vi "Channel Initialize.vi"(0 "Item Ref in":T2 format="%.0x", 7 "error in (no error)":errorcluster, 8 "Starting Address Ref in":refnum<vi>) -> (14 "Default Value":dbl, 16 "Radix":T1, 17 "Sub-Index (Bool)":u16, 18 "Registers":i32, 19 "input?":bool, 20 "Channel Ref out":T2 format="%.0x", 21 "Name":string, 22 "Description":string, 23 "Starting Address":u16, 24 "DataType":T3, 25 "Valid?":bool, 26 "Status Message":string, 27 "error out":errorcluster)   [LabVIEW 2019, in "Modbus Master System Explorer.lvlib"]
uses:
  Modbus Master System Explorer.lvlib
  Shared/Controls/Data Model/DataType.ctl
  <vilib>/NI VeriStand/Custom Device API/Custom Device Item Ref.ctl
  Radix.ctl
  <vilib>/NI VeriStand/Custom Device API/Custom Device API.lvlib
  Shared/Modbus Master Shared.lvlib
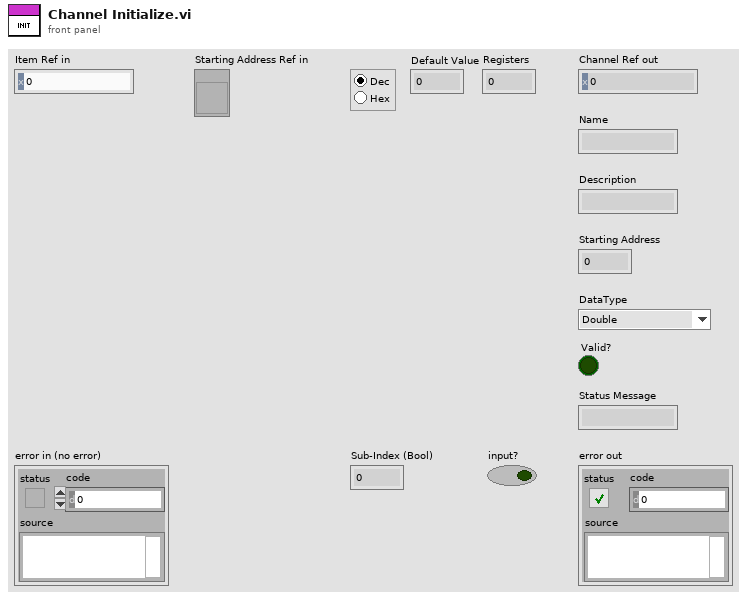
[diagram p1: front panel]
types:
  T1 = typedef "Modbus Master System Explorer.lvlib/Radix.ctl" = enum32{"Decimal", "Hexidecimal"}
  T2 = typedef "Custom Device API.lvlib/Custom Device Item Ref.ctl" = u64
  T3 = typedef "Modbus Master Shared.lvlib/DataType.ctl" = enum16{"Double", "Single", "I64", "I32", "I16", "I8", "U64", "U32", "U16", "U8", "Boolean"}
  T4 = typedef "Custom Device API.lvlib/Custom Device Item Info.ctl" = cluster{"Name":string, "Is Channel":bool, "GUID":string, "Is Waveform":bool}
  T5 = typedef "Modbus Master Shared.lvlib/Mapping.ctl" = cluster{"DataType":T3, "Starting Address":u16, "Sub-Index (Bool)":u16, "VS Reference":T2}
  T6 = typedef "Custom Device API.lvlib/Custom Device Channel.ctl" = cluster{"Type":T7, "Units":string, "Default Value":dbl, "Faultable":bool, "Scalable":bool}
  T7 = typedef "Custom Device API.lvlib/Custom Device Channel Type.ctl" = enum16{"Input", "Output"}
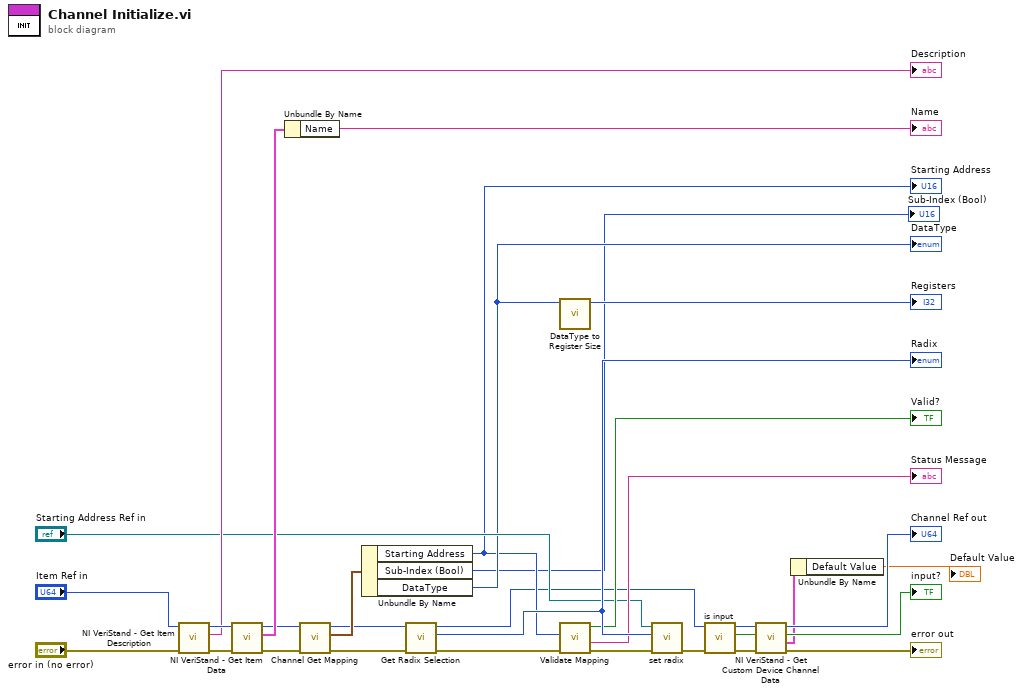
[diagram p0: block diagram]
diagram:
  n1 = call <vilib>:"NI VeriStand - Get Item Description.vi"("error in (no error)"="error in (no error)", "Item Ref in"="Item Ref in") -> ("error out"=w30:errorcluster, "Description"=→"Description":string, "Item Ref out"=w31:T2)  [unwired: 7 out]
  n2 = call <vilib>:"NI VeriStand - Get Item Data.vi"("error in (no error)"=w30, "Item Ref in"=w31) -> ("error out"=w27:errorcluster, "Item Info"=w29:T4, "Item Ref out"=w28:T2)  [unwired: 7 out]
  n3 = Unbundle By Name(w29) -> ("Name"=→"Name":string)
  n4 = call "Channel Get Mapping.vi"("error in (no error)"=w27, "Item Ref in"=w28) -> ("error out"=w24:errorcluster, "Mapping"=w26:T5, "Item Ref out"=w25:T2)  [unwired: 7 in]
  n5 = Unbundle By Name(w26) -> ("Starting Address"=w11:u16, "Sub-Index (Bool)"=→"Sub-Index (Bool)":u16, "DataType"=w12:T3)
  "Starting Address" <- w11
  "DataType" <- w12
  n6 = call "Get Radix Selection.vi"("error in (no error)"=w24, "Item Ref in"=w25) -> ("error out"=w23:errorcluster, "Radix"=w22:T1, "Item Ref out"=w9:T2)  [unwired: 7 in]
  "Radix" <- w22
  n7 = call "DataType to Register Size.vi"("DataType"=w12) -> ("Registers"=→"Registers":i32)  [unwired: 9 in, 1 out]
  n8 = call "Validate Mapping.vi"("error in (no error)"=w23, "Mapping"=w11) -> ("error out"=w21:errorcluster, "Status Message"=→"Status Message":string, "Valid?"=→"Valid?":bool)  [unwired: 7 in]
  n9 = call "set radix.vi"("error in (no error)"=w21, "Radix"=w22, "Digital in"="Starting Address Ref in") -> ("error out"=w10:errorcluster)  [unwired: 8 in]
  n10 = call "is input.vi"("error in (no error)"=w10, "Item Ref in"=w9) -> ("error out"=w5:errorcluster, "input?"=→"input?":bool, "Channel Ref out"=w6:T2)  [unwired: 7 in]
  n11 = call <vilib>:"NI VeriStand - Get Custom Device Channel Data.vi"("error in (no error)"=w5, "Channel Ref in"=w6) -> ("error out"=→"error out":errorcluster, "Channel"=w2:T6, "Channel Ref out"=→"Channel Ref out":T2)  [unwired: 4 in, 3 out]
  n12 = Unbundle By Name(w2) -> ("Default Value"=→"Default Value":dbl)
